vi "TP_Module.vi"   [LabVIEW 2012]
uses:
  Functional Global Variants/TP_GV_UI_Ref.vi
types:
  T1 = enum16{"Create Queue", "Get Queue", "Destory Queue"}
  T2 = typedef "TP_UI Ref.ctl" = cluster{"This VI":refnum<vi>, "String":refnum<vi>, "OK Button":refnum<vi>, "Stop Button":refnum<vi>}
  T3 = typedef "TP_Message Queue.lvlib/Message Cluster.ctl" = cluster{"Message":string, "Message Data":variant}
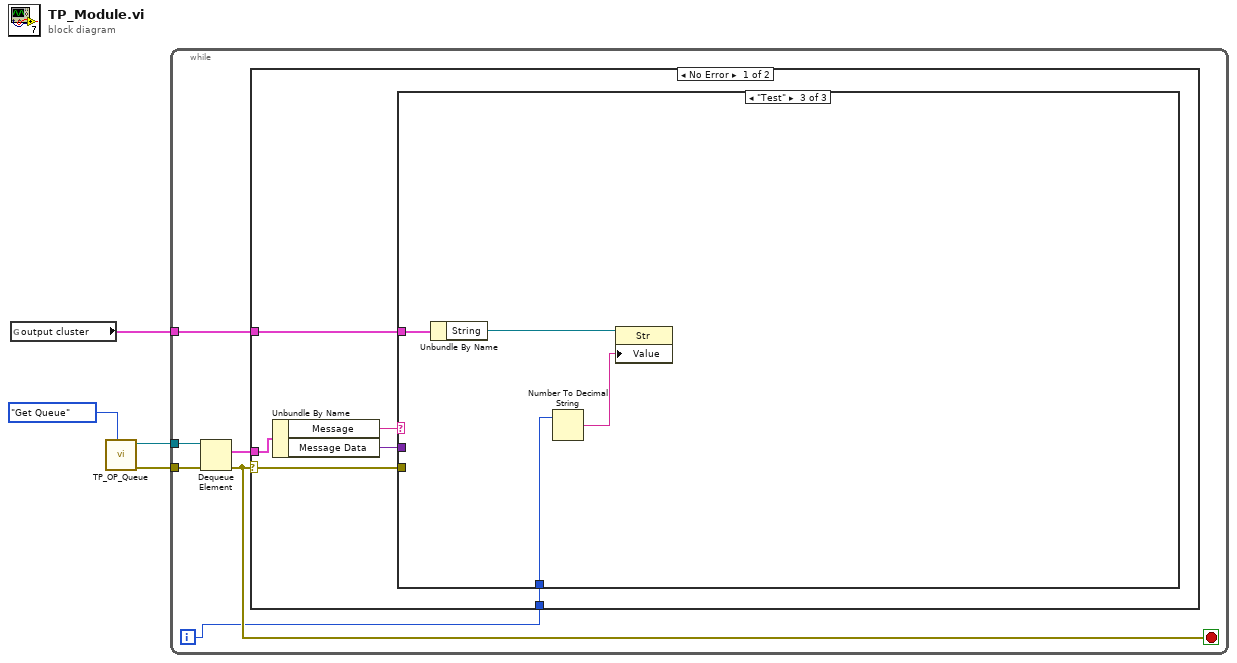
[diagram p0: block diagram]
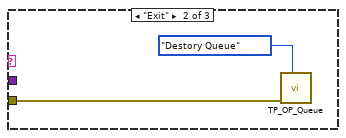
[diagram p3: hidden frame]
diagram:
  n1 = global read "TP_GV_UI_Ref.vi" "output cluster"() -> (w1:T2)
  n2 = call "TP_OP_Queue.vi"("OP_Queue (get queue)"=T1."Get Queue") -> ("error out"=w2:errorcluster, "queue out"=w3:refnum<queue>)  [unwired: 9 in]
  n3 = while {
    tunnel: w3 -> [w9]
    tunnel: w2 -> [w10]
    tunnel: w1 -> [w6]
    i -> [w5]
    stop <- w7 stop-if-true
    n4 = Dequeue Element(queue=w9, error in (no error)=w10) -> (element=w8:T3, error out=w7:errorcluster)  [unwired: 1 in, 2 out]
    n5 = case shown="No Error" w7 {
      selector: w7 -> [w15 _]
      tunnel: w8 -> [w16 _]
      tunnel: w6 -> [w12 _]
      tunnel: w5 -> [w11 _]
      frame No Error {
        n6 = Unbundle By Name(w16) -> ("Message"=w14:string, "Message Data"=w13:variant)
        n7 = case shown="\"Test\"" w14 {
          tunnel: w15 -> [_ w18 _]
          tunnel: w13 -> [_ _ _]
          tunnel: w12 -> [_ _ w22]
          tunnel: w11 -> [_ _ w19]
          frame "Nop", Default {
          }
          frame "Exit" {
            n8 = call "TP_OP_Queue.vi"("OP_Queue (get queue)"=T1."Destory Queue", "error in"=w18) -> ()  [unwired: 8 in, 2 out]
          }
          frame "Test" {
            n9 = Unbundle By Name(w22) -> ("String"=w21:refnum<vi>)
            n10 = Number To Decimal String(number=w19) -> (decimal integer string=w20:string)  [unwired: 1 in]
            n11 = property class="Str"(reference=w21, "Value"=w20) -> ()  [unwired: 1 in, 2 out]
          }
        }
      }
      frame Error {
      }
    }
  }
